vi "PNA fetch calkit.vi"() -> ()   [LabVIEW 2020]
panel:
  out "read buffer 2":string
  out "read buffer":string
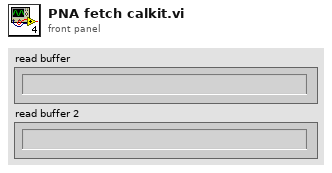
[diagram p1: front panel]
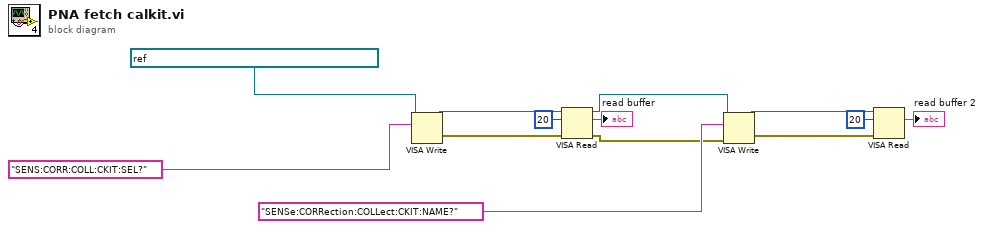
[diagram p0: block diagram]
diagram:
  n1 = VISA Write(VISA resource name=refnum<visa-resource-name> "USB0::0x0957::0x0118::MY52221020::INSTR", write buffer="SENS:CORR:COLL:CKIT:SEL?") -> (VISA resource name out=w13:refnum<visa-resource-name>, error out=w12:errorcluster)  [unwired: 1 in, 1 out]
  n2 = VISA Read(VISA resource name=w13, byte count=u32 20, error in (no error)=w12) -> (VISA resource name out=w5:refnum<visa-resource-name>, read buffer=→"read buffer":string, error out=w6:errorcluster)  [unwired: 1 out]
  n3 = VISA Write(VISA resource name=w5, write buffer="SENSe:CORRection:COLLect:CKIT:NAME?", error in (no error)=w6) -> (VISA resource name out=w7:refnum<visa-resource-name>, error out=w8:errorcluster)  [unwired: 1 out]
  n4 = VISA Read(VISA resource name=w7, byte count=u32 20, error in (no error)=w8) -> (read buffer=→"read buffer 2":string)  [unwired: 3 out]
